vi "Read incoming label data.vi"(8 "error in (no error)":errorcluster, 11 "Driver Data":T1 {"Num Bits" min=1 max=32; "Start Bit" min=8 max=31}) -> (0 "error out":errorcluster, 3 "Values":dbl[](array[numeric]))   [LabVIEW 2011, in "AIT 1553 Custom Device.lvlib"]
uses:
  AIT 1553 Custom Device.lvlib
  RT Controls/Driver Data.ctl
  Controls and Global/Start Bit.ctl
  Controls and Global/Number of Bits.ctl
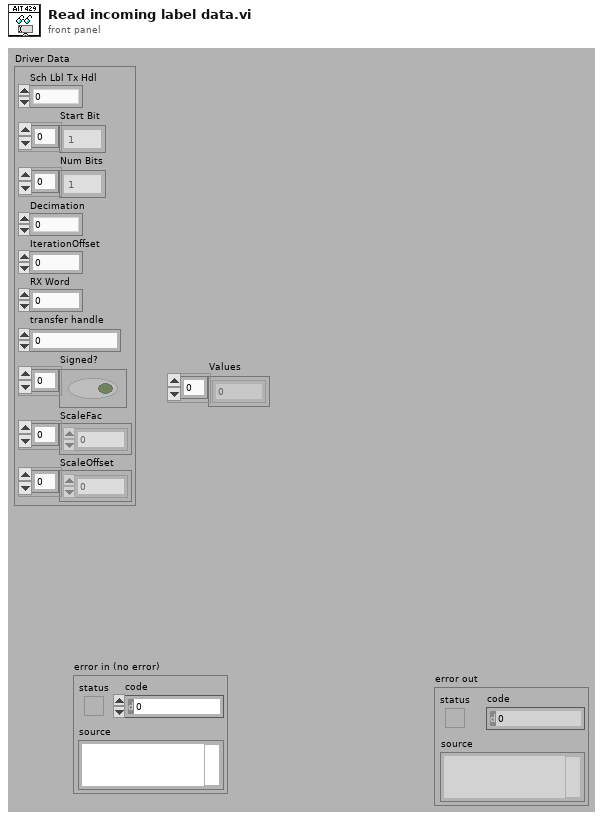
[diagram p1: front panel]
types:
  T1 = typedef "AIT 1553 Custom Device.lvlib/Driver Data.ctl" = cluster{"Sch Lbl Tx Hdl":u32, "Start Bit":T2[], "Num Bits":T3[], "Decimation":i32, "IterationOffset":i32, "RX Word":u32, "transfer handle":u32, "Signed?":bool[], "ScaleFac":dbl[], "ScaleOffset":dbl[]}
  T2 = typedef "AIT 1553 Custom Device.lvlib/Start Bit.ctl" = i32
  T3 = typedef "AIT 1553 Custom Device.lvlib/Number of Bits.ctl" = i32
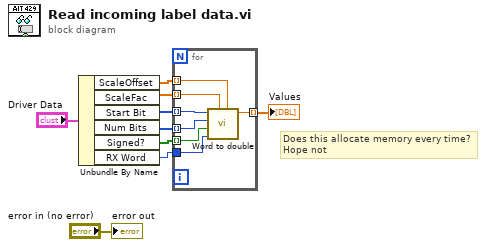
[diagram p0: block diagram]
diagram:
  # "Does this allocate memory every time?\nHope not"
  n1 = Unbundle By Name("Driver Data") -> ("ScaleOffset"=w1:dbl[], "ScaleFac"=w2:dbl[], "Start Bit"=w3:T2[], "Num Bits"=w4:T3[], "Signed?"=w5:bool[], "RX Word"=w6:u32)
  n2 = for {
    tunnel: [w16] -> w7 mode=indexing
    tunnel: w6 -> [w15]
    tunnel: w5 -> [w14] mode=indexing
    tunnel: w4 -> [w13] mode=indexing
    tunnel: w3 -> [w12] mode=indexing
    tunnel: w2 -> [w11] mode=indexing
    tunnel: w1 -> [w10] mode=indexing
    n3 = call "Word to double.vi"("ScaleOffset (0)"=w10, "ScaleFac (1)"=w11, "word"=w15, "Signed? (F)"=w14, "Number of Bits"=w13, "Start Bit"=w12) -> ("Double"=w16:dbl)  [unwired: 5 in]
  }
  "Values" <- w7
  "error out" <- "error in (no error)"
